vi "Create RDB Cluster.vi"(7 "datalog path":path=path "C:/Users/admin/Desktop/datalog.txt", 8 "error out":errorcluster, 11 "Channel Refs":T4[](array[typedef]) format="%.0x") -> (0 "error out 2":errorcluster, 3 "Array":T1)   [LabVIEW 2023, in "Vires VTD System Explorer.lvlib"]
uses:
  Vires VTD System Explorer.lvlib
  <vilib>/NI VeriStand/Custom Device API/Custom Device Item Ref.ctl
  RDB Data.ctl
  RDB/RDB Object.ctl
  RDB/RDB Player Object.ctl
  <vilib>/NI VeriStand/Custom Device API/Get Item Property (Variant).vi
  <vilib>/Utility/xml.llb/Write to XML File(string).vi
  RDB/RDB.lvlib
  <vilib>/NI VeriStand/Custom Device API/Custom Device API.lvlib
  Shared/Vires VTD Shared.lvlib
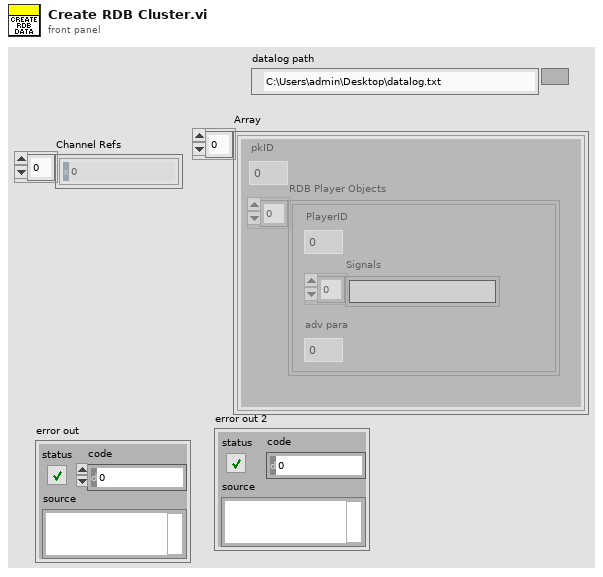
[diagram p1: front panel]
types:
  T1 = typedef "Vires VTD Shared.lvlib/RDB Data.ctl" = T2[]
  T2 = typedef "RDB.lvlib/RDB Object.ctl" = cluster{"pkID":i32, "RDB Player Objects":T3[]}
  T3 = typedef "RDB.lvlib/RDB Player Object.ctl" = cluster{"PlayerID":i32, "Signals":string[], "adv para":i32}
  T4 = typedef "Custom Device API.lvlib/Custom Device Item Ref.ctl" = u64
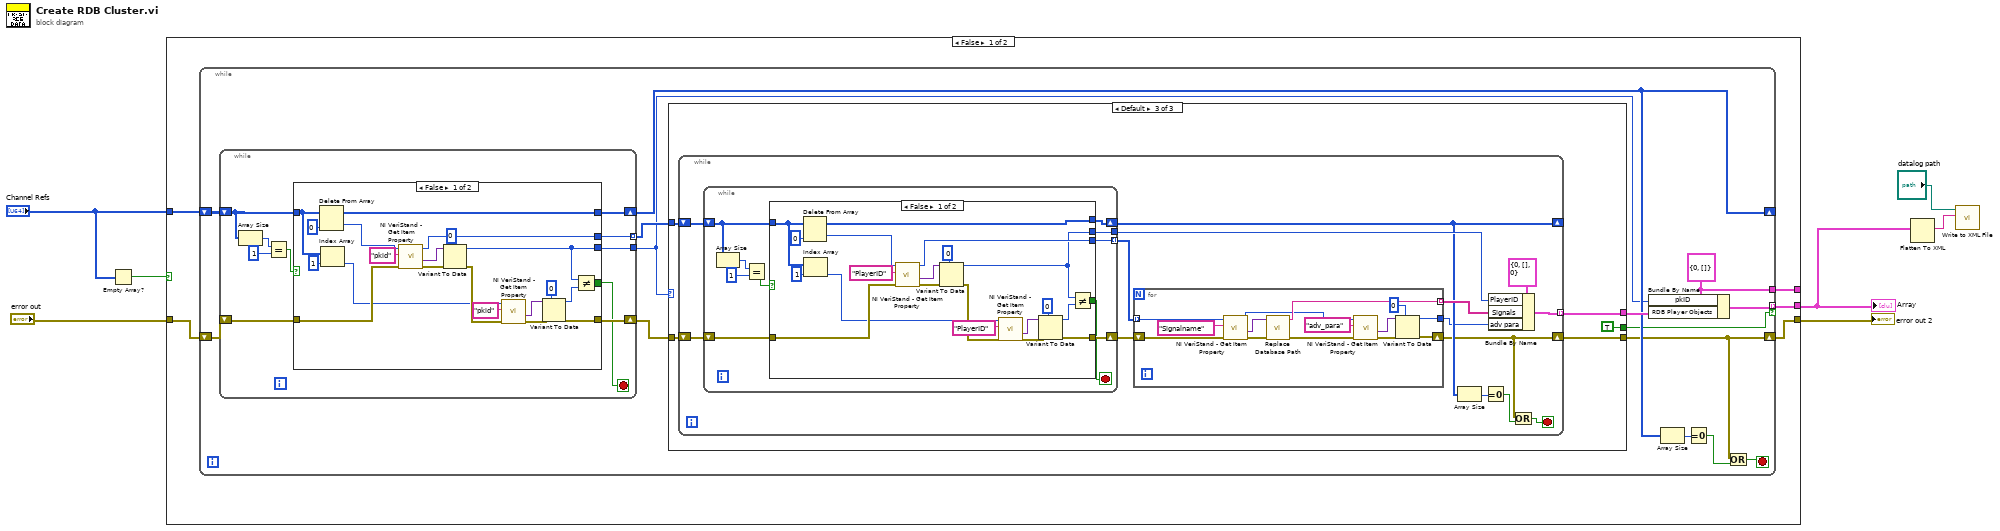
[diagram p0: block diagram]
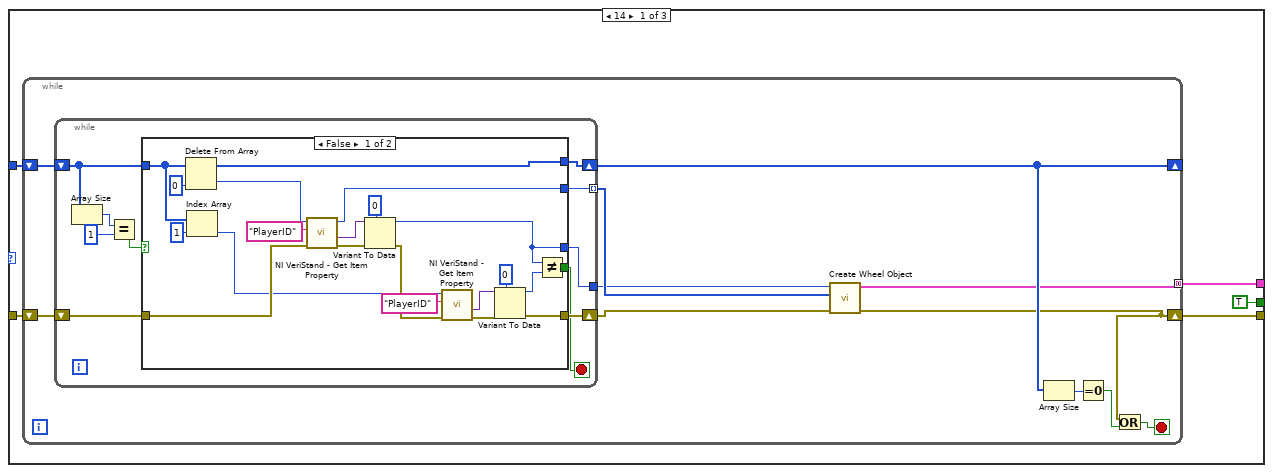
[diagram p2: hidden frame]
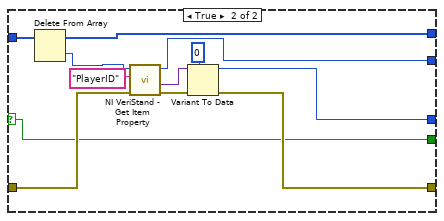
[diagram p3: hidden frame]
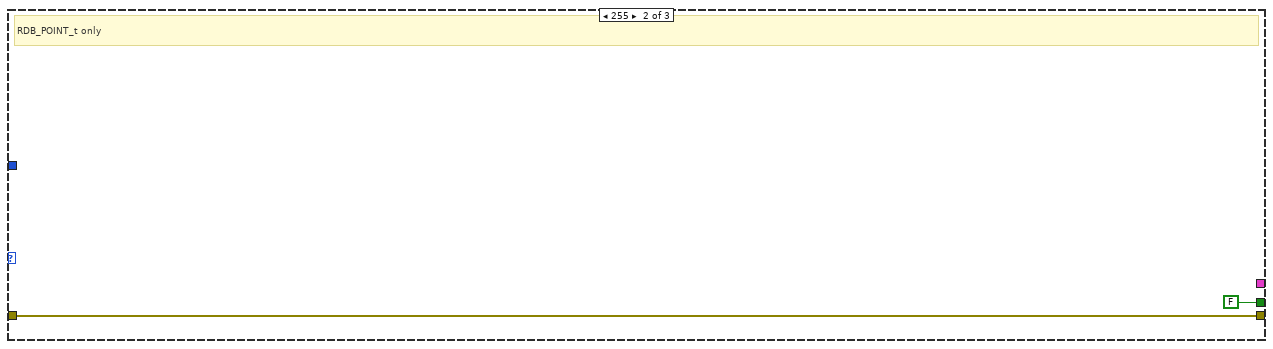
[diagram p4: hidden frame]
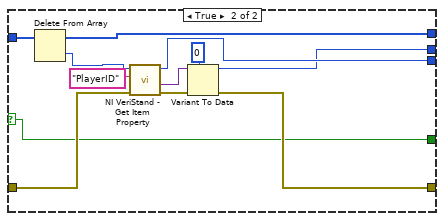
[diagram p5: hidden frame]
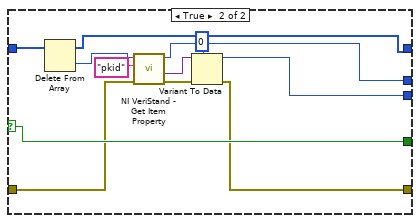
[diagram p6: hidden frame]
diagram:
  n1 = Empty Array?(array="Channel Refs") -> (empty?=w4:bool)
  n2 = case shown="False" w4 {
    tunnel: "Channel Refs" -> [w12 _]
    tunnel: "error out" -> [w11 w207]
    tunnel: [w10 w207] -> w6
    tunnel: [w9 _] -> w2
    tunnel: [w8 _] -> _
    frame False {
      n3 = while {
        shift-right: [w18] -> _
        shift-left: w12 -> [w26]
        shift-right: [w17] -> w10
        shift-left: w11 -> [w22]
        tunnel: [w16] -> w9 mode=indexing if=w13
        tunnel: [w14] -> w8
        stop <- w19 stop-if-true
        w14 = T2 {"pkID"=0, "RDB Player Objects"=[]} ("RDB Object")
        n4 = while {
          shift-right: [w173] -> w25
          shift-left: w22 -> [w172]
          tunnel: [w170] -> w24 mode=indexing
          tunnel: [w169] -> w15
          shift-right: [w168] -> w18
          shift-left: w26 -> [w167]
          stop <- w171 stop-if-true
          n5 = Array Size(array=w167) -> (size(s)=w166:i32)
          n6 = Equal?(x=w166, y=1) -> (x = y?=w164:bool)
          n7 = case shown="False" w164 {
            selector: w164 -> [_ w206]
            tunnel: [w187 w199] -> w173
            tunnel: w172 -> [w186 w200]
            tunnel: [w182 w206] -> w171
            tunnel: [w181 w197] -> w170
            tunnel: [w180 w198] -> w169
            tunnel: [w176 w195] -> w168
            tunnel: w167 -> [w174 w196]
            frame False {
              n8 = Delete From Array(array=w174, index=0) -> (deleted portion=w177:T4, array with subset deleted=w176:T4[])  [unwired: 1 in]
              n9 = Index Array(array=w174, index=1) -> (element=w175:T4)
              n10 = call-poly <vilib>:"NI VeriStand - Get Item Property.vi"("error in (no error)"=w186, "Property Name"="pkid", "Item Ref in"=w177) -> ("error out"=w192:errorcluster, "Value"=w191:variant, "Item Ref out"=w181:T4)  [unwired: 5 in, 1 out]
              n11 = Variant To Data(error in=w192, type=u8 0, Variant=w191) -> (data=w180:u8, error out=w190:errorcluster)
              n12 = call-poly <vilib>:"NI VeriStand - Get Item Property.vi"("error in (no error)"=w190, "Property Name"="pkid", "Item Ref in"=w175) -> ("error out"=w189:errorcluster, "Value"=w188:variant)  [unwired: 5 in, 2 out]
              n13 = Variant To Data(error in=w189, type=u8 0, Variant=w188) -> (data=w184:u8, error out=w187:errorcluster)
              n14 = Not Equal?(x=w180, y=w184) -> (x != y?=w182:bool)
            }
            frame True {
              n15 = Delete From Array(array=w196) -> (deleted portion=w201:T4, array with subset deleted=w195:T4[])  [unwired: 2 in]
              n16 = call-poly <vilib>:"NI VeriStand - Get Item Property.vi"("error in (no error)"=w200, "Property Name"="pkid", "Item Ref in"=w201) -> ("error out"=w204:errorcluster, "Value"=w203:variant, "Item Ref out"=w197:T4)  [unwired: 5 in, 1 out]
              n17 = Variant To Data(error in=w204, type=u8 0, Variant=w203) -> (data=w198:u8, error out=w199:errorcluster)
            }
          }
        }
        n18 = case shown="Default" w15 {
          tunnel: w25 -> [w30 w87 w92]
          tunnel: w24 -> [w31 _ w91]
          tunnel: [w29 _ w90] -> w23
          tunnel: [w28 w87 w89] -> w17
          tunnel: [TRUE FALSE TRUE] -> w13
          frame 14 {
            n19 = while {
              shift-right: [w37] -> _
              shift-left: w31 -> [w41]
              shift-right: [w33] -> w28
              shift-left: w30 -> [w42]
              tunnel: [w32] -> w29 mode=concatenating
              stop <- w36 stop-if-true
              n20 = while {
                shift-right: [w52] -> w39
                shift-left: w42 -> [w51]
                tunnel: [w49] -> w40 mode=indexing
                tunnel: [w48] -> w38
                shift-right: [w43] -> w37
                shift-left: w41 -> [w45]
                stop <- w50 stop-if-true
                n21 = Array Size(array=w45) -> (size(s)=w46:i32)
                n22 = Equal?(x=w46, y=1) -> (x = y?=w44:bool)
                n23 = case shown="False" w44 {
                  selector: w44 -> [_ w79]
                  tunnel: [w66 w80] -> w52
                  tunnel: w51 -> [w65 w81]
                  tunnel: [w61 w79] -> w50
                  tunnel: [w60 w78] -> w49
                  tunnel: [w59 w77] -> w48
                  tunnel: w45 -> [w58 w76]
                  tunnel: [w53 w75] -> w43
                  frame False {
                    n24 = Delete From Array(array=w58, index=0) -> (deleted portion=w54:T4, array with subset deleted=w53:T4[])  [unwired: 1 in]
                    n25 = Index Array(array=w58, index=1) -> (element=w57:T4)
                    n26 = call-poly <vilib>:"NI VeriStand - Get Item Property.vi"("error in (no error)"=w65, "Property Name"="PlayerID", "Item Ref in"=w54) -> ("error out"=w71:errorcluster, "Value"=w70:variant, "Item Ref out"=w60:T4)  [unwired: 5 in, 1 out]
                    n27 = Variant To Data(error in=w71, type=u8 0, Variant=w70) -> (data=w59:u8, error out=w69:errorcluster)
                    n28 = call-poly <vilib>:"NI VeriStand - Get Item Property.vi"("error in (no error)"=w69, "Property Name"="PlayerID", "Item Ref in"=w57) -> ("error out"=w68:errorcluster, "Value"=w67:variant)  [unwired: 5 in, 2 out]
                    n29 = Variant To Data(error in=w68, type=u8 0, Variant=w67) -> (data=w63:u8, error out=w66:errorcluster)
                    n30 = Not Equal?(x=w59, y=w63) -> (x != y?=w61:bool)
                  }
                  frame True {
                    n31 = Delete From Array(array=w76) -> (deleted portion=w74:T4, array with subset deleted=w75:T4[])  [unwired: 2 in]
                    n32 = call-poly <vilib>:"NI VeriStand - Get Item Property.vi"("error in (no error)"=w81, "Property Name"="PlayerID", "Item Ref in"=w74) -> ("error out"=w83:errorcluster, "Value"=w84:variant, "Item Ref out"=w78:T4)  [unwired: 5 in, 1 out]
                    n33 = Variant To Data(error in=w83, type=u8 0, Variant=w84) -> (data=w77:u8, error out=w80:errorcluster)
                  }
                }
              }
              n34 = call "Create Wheel Object.vi"("error out 2"=w39, "Array"=w40, "Numeric"=w38) -> ("error out"=w33:errorcluster, "Array 2"=w32:T3[])  [unwired: 7 in]
              n35 = Array Size(array=w37) -> (size(s)=w35:i32)
              n36 = Equal To 0?(x=w35) -> (x = 0?=w34:bool)
              n37 = Or(x=w33, y=w34) -> (x .or. y?=w36:bool)
            }
          }
          frame 255 {
            # "RDB_POINT_t only"
          }
          frame Default {
            n38 = while {
              shift-right: [w99] -> _
              shift-left: w91 -> [w105]
              shift-right: [w95] -> w89
              shift-left: w92 -> [w106]
              tunnel: [w94] -> w90 mode=indexing
              stop <- w98 stop-if-true
              n39 = while {
                shift-right: [w116] -> w103
                shift-left: w106 -> [w115]
                tunnel: [w113] -> w104 mode=indexing
                tunnel: [w112] -> w101
                shift-right: [w107] -> w99
                shift-left: w105 -> [w109]
                stop <- w114 stop-if-true
                n40 = Array Size(array=w109) -> (size(s)=w110:i32)
                n41 = Equal?(x=w110, y=1) -> (x = y?=w108:bool)
                n42 = case shown="False" w108 {
                  selector: w108 -> [_ w143]
                  tunnel: [w130 w144] -> w116
                  tunnel: w115 -> [w129 w145]
                  tunnel: [w125 w143] -> w114
                  tunnel: [w124 w142] -> w113
                  tunnel: [w123 w141] -> w112
                  tunnel: w109 -> [w122 w140]
                  tunnel: [w117 w139] -> w107
                  frame False {
                    n43 = Delete From Array(array=w122, index=0) -> (deleted portion=w118:T4, array with subset deleted=w117:T4[])  [unwired: 1 in]
                    n44 = Index Array(array=w122, index=1) -> (element=w121:T4)
                    n45 = call-poly <vilib>:"NI VeriStand - Get Item Property.vi"("error in (no error)"=w129, "Property Name"="PlayerID", "Item Ref in"=w118) -> ("error out"=w135:errorcluster, "Value"=w134:variant, "Item Ref out"=w124:T4)  [unwired: 5 in, 1 out]
                    n46 = Variant To Data(error in=w135, type=u8 0, Variant=w134) -> (data=w123:u8, error out=w133:errorcluster)
                    n47 = call-poly <vilib>:"NI VeriStand - Get Item Property.vi"("error in (no error)"=w133, "Property Name"="PlayerID", "Item Ref in"=w121) -> ("error out"=w132:errorcluster, "Value"=w131:variant)  [unwired: 5 in, 2 out]
                    n48 = Variant To Data(error in=w132, type=u8 0, Variant=w131) -> (data=w127:u8, error out=w130:errorcluster)
                    n49 = Not Equal?(x=w123, y=w127) -> (x != y?=w125:bool)
                  }
                  frame True {
                    n50 = Delete From Array(array=w140) -> (deleted portion=w138:T4, array with subset deleted=w139:T4[])  [unwired: 2 in]
                    n51 = call-poly <vilib>:"NI VeriStand - Get Item Property.vi"("error in (no error)"=w145, "Property Name"="PlayerID", "Item Ref in"=w138) -> ("error out"=w147:errorcluster, "Value"=w148:variant, "Item Ref out"=w142:T4)  [unwired: 5 in, 1 out]
                    n52 = Variant To Data(error in=w147, type=u8 0, Variant=w148) -> (data=w141:u8, error out=w144:errorcluster)
                  }
                }
              }
              n53 = for {
                tunnel: w104 -> [w159] mode=indexing
                shift-right: [w153] -> w95
                shift-left: w103 -> [w160]
                tunnel: [w158] -> w102 mode=indexing
                tunnel: [w150] -> w93
                n54 = call-poly <vilib>:"NI VeriStand - Get Item Property.vi"("error in (no error)"=w160, "Property Name"="Signalname", "Item Ref in"=w159) -> ("error out"=w162:errorcluster, "Value"=w163:variant, "Item Ref out"=w156:T4)  [unwired: 5 in, 1 out]
                n55 = call "Replace Database Path.vi"("error in (no error)"=w162, "Value"=w163) -> ("error out"=w157:errorcluster, "Property Name"=w158:string)  [unwired: 8 in]
                n56 = call-poly <vilib>:"NI VeriStand - Get Item Property.vi"("error in (no error)"=w157, "Property Name"="adv_para", "Item Ref in"=w156) -> ("error out"=w154:errorcluster, "Value"=w151:variant)  [unwired: 5 in, 2 out]
                n57 = Variant To Data(error in=w154, type=u8 0, Variant=w151) -> (data=w150:u8, error out=w153:errorcluster)
              }
              n58 = Array Size(array=w99) -> (size(s)=w97:i32)
              n59 = Equal To 0?(x=w97) -> (x = 0?=w96:bool)
              n60 = Bundle By Name(cluster=T3 {"PlayerID"=0, "Signals"=[], "adv para"=0} ("RDB Player Objects"), "PlayerID"=w101, "Signals"=w102, "adv para"=w93) -> (w94:T3)
              n61 = Or(x=w95, y=w96) -> (x .or. y?=w98:bool)
            }
          }
        }
        n62 = Bundle By Name(cluster=w14, "pkID"=w15, "RDB Player Objects"=w23) -> (w16:T2)
        n63 = Array Size(array=w18) -> (size(s)=w20:i32)
        n64 = Equal To 0?(x=w20) -> (x = 0?=w21:bool)
        n65 = Or(x=w17, y=w21) -> (x .or. y?=w19:bool)
      }
    }
    frame True {
    }
  }
  "Array" <- w2
  "error out 2" <- w6
  n66 = Flatten To XML(6:w2) -> (2:w1:string)
  n67 = call-poly <vilib>:"Write to XML File.vi"("XML Input"=w1, "XML File Path"="datalog path") -> ()  [unwired: 7 in, 3 out]
